vi "Lidar.vi"(1 "read buffer":string) -> (0 "输出簇":T1)   [LabVIEW 2014]
panel:
  out "16位整型 2":u16
  out "16位整型":u16
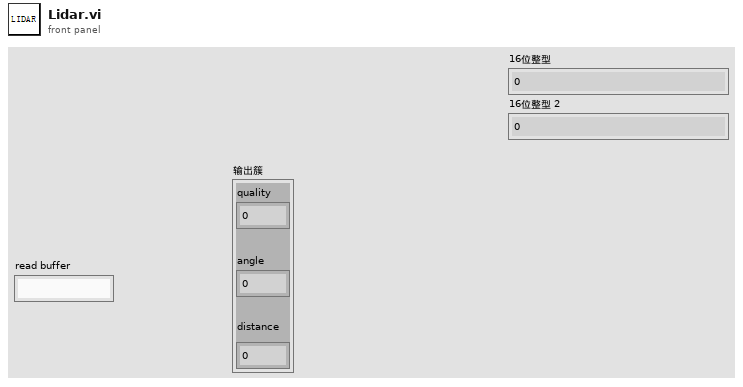
[diagram p1: front panel]
types:
  T1 = cluster{"quality":u8, "angle":u16, "distance\n":u16}
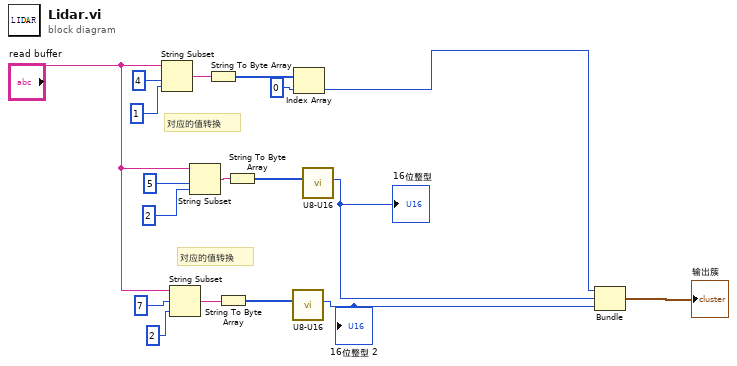
[diagram p0: block diagram]
diagram:
  # "对应的值转换"
  # "对应的值转换"
  n1 = String Subset(string="read buffer", offset (0)=4 ("长度（剩余）"), length (rest)=1 ("长度（剩余）")) -> (substring=w15:string)
  n2 = String Subset(string="read buffer", offset (0)=7 ("长度（剩余）"), length (rest)=2 ("长度（剩余）")) -> (substring=w18:string)
  n3 = String Subset(string="read buffer", offset (0)=5 ("长度（剩余）"), length (rest)=2 ("长度（剩余）")) -> (substring=w7:string)
  n4 = String To Byte Array(string=w15) -> (unsigned byte array=w11:u8[])
  n5 = String To Byte Array(string=w18) -> (unsigned byte array=w8:u8[])
  n6 = String To Byte Array(string=w7) -> (unsigned byte array=w2:u8[])
  n7 = call "U8-U16.vi"("数组"=w8) -> ("16位整型"=w3:u16)  [unwired: 8 in, 1 out]
  "16位整型 2" <- w3
  n8 = Index Array(array=w11, index=0 ("索引")) -> (element=w9:u8)
  n9 = call "U8-U16.vi"("数组"=w2) -> ("16位整型"=w1:u16)  [unwired: 8 in, 1 out]
  "16位整型" <- w1
  n10 = Bundle(w9, "16位整型"=w1, "16位整型"=w3) -> (→"输出簇":cluster{u8, "16位整型":u16, "16位整型":u16})  [unwired: 1 in]
